vi "_PC_NS_Signal_Execution.vi"(0 "SysMsg":refnum<vi>, 1 "Network\nstream":refnum<vi>, 3 "Stop":refnum<vi>, 5 "# signal in NS":refnum<vi>, 11 "error in (no error)":errorcluster, 12 "Sig Queue":refnum<queue>, 14 "Conn_Bool":refnum<data-value>) -> ()   [LabVIEW 2018]
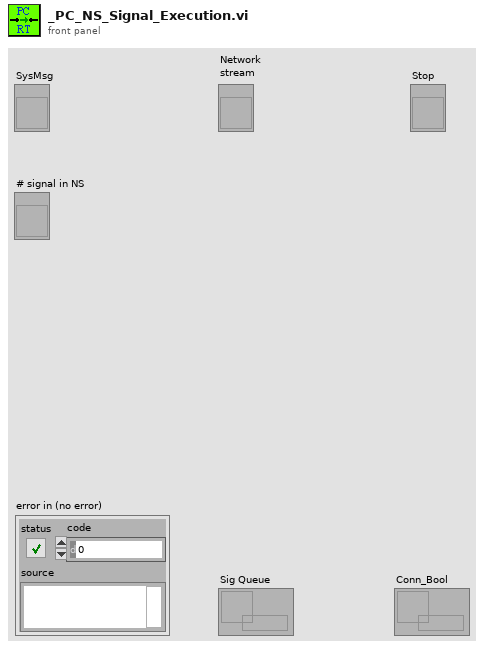
[diagram p1: front panel]
types:
  T1 = enum8{"Enabled", "Disabled", "Disabled and Grayed Out"}
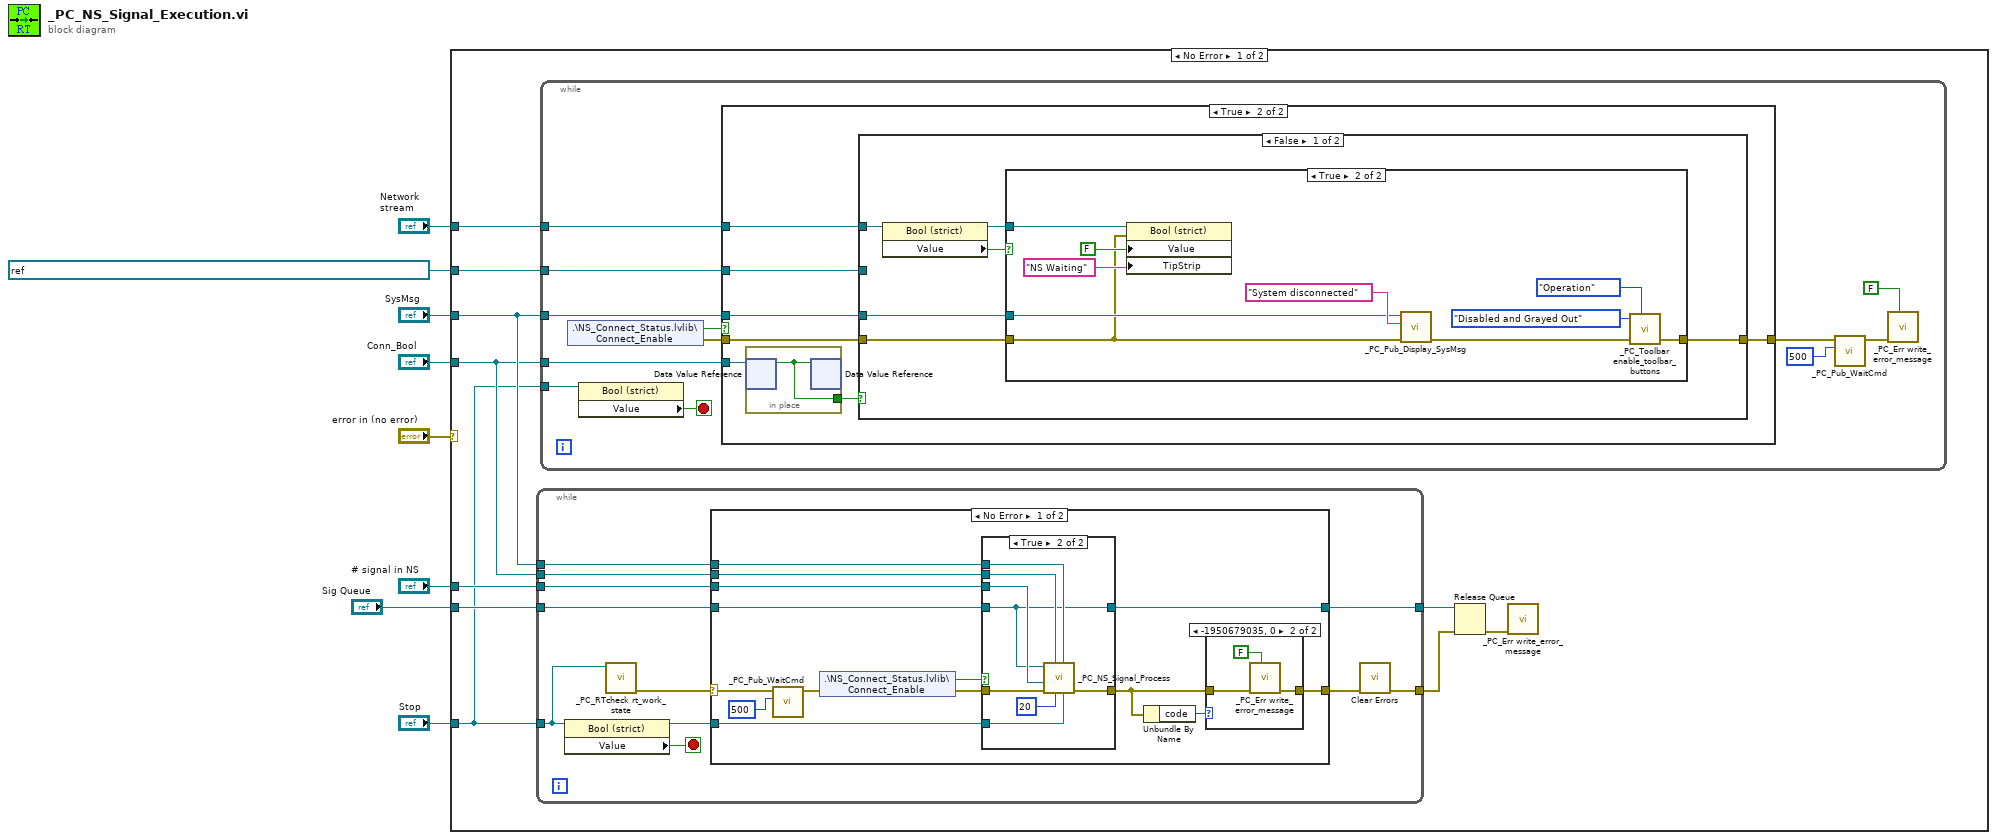
[diagram p0: block diagram]
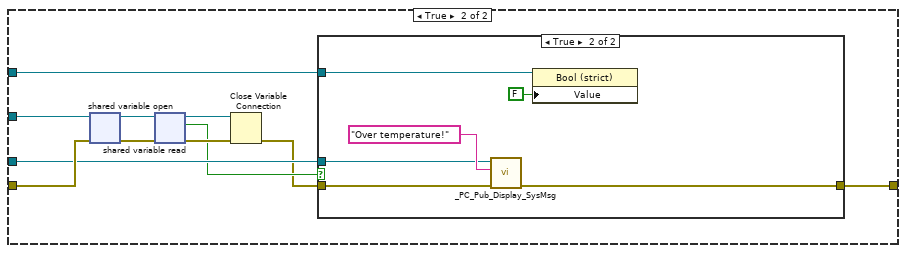
[diagram p4: hidden frame]
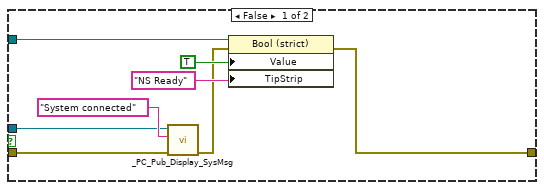
[diagram p5: hidden frame]
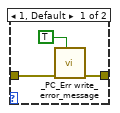
[diagram p6: hidden frame]
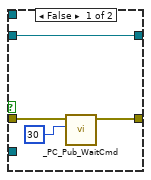
[diagram p7: hidden frame]
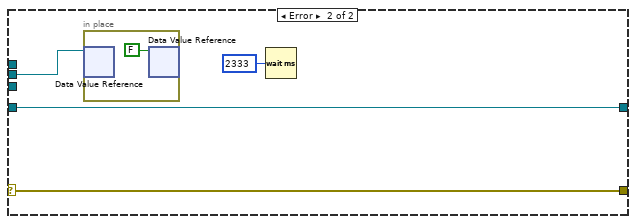
[diagram p8: hidden frame]
diagram:
  n1 = case shown="No Error" "error in (no error)" {
    tunnel: "# signal in NS" -> [w18 _]
    tunnel: "Network\nstream" -> [w17 _]
    tunnel: "SysMsg" -> [w16 _]
    tunnel: "Conn_Bool" -> [w15 _]
    tunnel: "Sig Queue" -> [w14 _]
    tunnel: refnum<k21> "ni.var.psp://NI-sbRIO/_RT_CtrlLoop_Safty_Variables/OverTemperature" ("shared variable refnum in") -> [w13 _]
    tunnel: "Stop" -> [w12 _]
    frame No Error {
      n2 = while {
        tunnel: w18 -> [w92]
        tunnel: w14 -> [w86]
        tunnel: w16 -> [w91]
        tunnel: w15 -> [w90]
        tunnel: w12 -> [w87]
        tunnel: [w85] -> w11
        tunnel: [w83] -> w10
        stop <- w89 stop-if-true
        n3 = property class="Bool (strict)"(reference=w87) -> (reference out=w82:refnum<vi>, "Value"=w89:bool)  [unwired: 1 in, 1 out]
        n4 = call "_PC_RTcheck rt_work_state.vi"("Stop"=w87) -> ("error out"=w88:errorcluster)  [unwired: 10 in]
        n5 = case shown="No Error" w88 {
          selector: w88 -> [w97 w126]
          tunnel: w92 -> [w106 _]
          tunnel: w91 -> [w103 _]
          tunnel: w90 -> [w102 w128]
          tunnel: [w94 w126] -> w84
          tunnel: w86 -> [w96 w125]
          tunnel: [w95 w125] -> w85
          tunnel: w82 -> [w93 _]
          frame No Error {
            n6 = call "_PC_Pub_WaitCmd.vi"("milliseconds to wait"=u32 500, "error in (no error)"=w97) -> ("error out"=w100:errorcluster)  [unwired: 9 in]
            n7 = shared-variable ".\\NS_Connect_Status.lvlib\\Connect_Enable"(error in=w100) -> (w104:bool, error out=w105:errorcluster)
            n8 = case shown="True" w104 {
              tunnel: w105 -> [w115 w123]
              tunnel: w106 -> [_ w122]
              tunnel: w96 -> [w113 w118]
              tunnel: [w114 w121] -> w98
              tunnel: w103 -> [_ w120]
              tunnel: w102 -> [_ w119]
              tunnel: [w113 w118] -> w95
              tunnel: w93 -> [_ w117]
              frame False {
                n9 = call "_PC_Pub_WaitCmd.vi"("milliseconds to wait"=u32 30, "error in (no error)"=w115) -> ("error out"=w114:errorcluster)  [unwired: 9 in]
              }
              frame True {
                n10 = call "_PC_NS_Signal_Process.vi"("Stop"=w117, "SysMsg"=w120, "Maximum Reader"=20, "Conn_Bool"=w119, "error in (no error)"=w123, "# signal in NS ref"=w122, "Sig Queue"=w118) -> ("error out"=w121:errorcluster)  [unwired: 4 in]
              }
            }
            n11 = Unbundle By Name(w98) -> ("code"=w99:i32)
            n12 = case shown="-1950679035, 0" w99 {
              tunnel: w98 -> [w108 w111]
              tunnel: [w107 w110] -> w94
              frame 1, Default {
                n13 = call "_PC_Err write_error_message.vi"("show msg( T )"=TRUE, "error in"=w108) -> ("error out"=w107:errorcluster)  [unwired: 9 in]
              }
              frame -1950679035, 0 {
                n14 = call "_PC_Err write_error_message.vi"("show msg( T )"=FALSE, "error in"=w111) -> ("error out"=w110:errorcluster)  [unwired: 9 in]
              }
            }
          }
          frame Error {
            n15 = in-place {
              n16 = in-place-dvr #1(w128) -> ()  [unwired: 2 out]
              n17 = in-place-dvr #1(FALSE ("data value")) -> ()  [unwired: 2 out]
            }
            n18 = Wait (ms)(milliseconds to wait=u32 2333) -> ()  [unwired: 1 out]
          }
        }
        n19 = call <vilib>:"Clear Errors.vi"("error in (no error)"=w84) -> ("error out"=w83:errorcluster)  [unwired: 5 in, 1 out]
      }
      n20 = while {
        tunnel: w16 -> [w29]
        tunnel: w17 -> [w28]
        tunnel: w15 -> [w27]
        tunnel: w13 -> [w22]
        tunnel: w12 -> [w20]
        stop <- w19 stop-if-true
        n21 = shared-variable ".\\NS_Connect_Status.lvlib\\Connect_Enable"() -> (w30:bool, error out=w26:errorcluster)  [unwired: 1 in]
        n22 = property class="Bool (strict)"(reference=w20) -> ("Value"=w19:bool)  [unwired: 1 in, 2 out]
        n23 = case shown="True" w30 {
          tunnel: w29 -> [_ w38]
          tunnel: w28 -> [_ w37]
          tunnel: [w31 w36] -> w24
          tunnel: w27 -> [_ w35]
          tunnel: w26 -> [w31 w33]
          tunnel: w22 -> [_ w32]
          frame False {
          }
          frame True {
            n24 = in-place {
              in-place-border: [w39] -> w34
              n25 = in-place-dvr #2(w35) -> (w39:bool)  [unwired: 1 out]
              n26 = in-place-dvr #2(w39) -> ()  [unwired: 2 out]
            }
            n27 = case shown="False" w34 {
              tunnel: w37 -> [w43 w63]
              tunnel: w33 -> [w45 w67]
              tunnel: [w44 w65] -> w36
              tunnel: w38 -> [w40 w66]
              tunnel: w32 -> [_ w64]
              frame False {
                n28 = property class="Bool (strict)"(reference=w43) -> (reference out=w41:refnum<vi>, "Value"=w42:bool)  [unwired: 1 in, 1 out]
                n29 = case shown="True" w42 {
                  tunnel: w45 -> [w46 w47]
                  tunnel: [w46 w48] -> w44
                  tunnel: w41 -> [_ w54]
                  tunnel: w40 -> [_ w49]
                  frame False {
                  }
                  frame True {
                    n30 = property class="Bool (strict)"(reference=w54, error in=w47, "Value"=FALSE, "TipStrip"="NS Waiting" ("Tip Strip")) -> ()  [unwired: 2 out]
                    n31 = call "_PC_Pub_Display_SysMsg.vi"("error in (no error)"=w47, "Msg String"="System disconnected" ("Msg in"), "SysMsg Ref In"=w49) -> ("error out"=w51:errorcluster)  [unwired: 7 in, 1 out]
                    n32 = call "_PC_Toolbar enable_toolbar_buttons.vi"("Disabled"=T1."Disabled and Grayed Out", "Function"=enum16{"Save reference", "Operation"}."Operation", "error in (no error)"=w51) -> ("error out"=w48:errorcluster)  [unwired: 6 in]
                  }
                }
              }
              frame True {
                n33 = shared-variable-open(w64, w67) -> (w59:refnum<k21>, w62:errorcluster)
                n34 = shared-variable-read(w59, w62) -> (w60:refnum<k21>, w61:errorcluster, w58:bool)
                n35 = Close Variable Connection(8:w61, 11:w60) -> (0:w57:errorcluster)
                n36 = case shown="True" w58 {
                  tunnel: w57 -> [w71 w80]
                  tunnel: [w68 w79] -> w65
                  tunnel: w66 -> [w70 w78]
                  tunnel: w63 -> [w69 w77]
                  frame False {
                    n37 = call "_PC_Pub_Display_SysMsg.vi"("error in (no error)"=w71, "Msg String"="System connected" ("Msg in"), "SysMsg Ref In"=w70) -> ("error out"=w72:errorcluster)  [unwired: 7 in, 1 out]
                    n38 = property class="Bool (strict)"(reference=w69, error in=w72, "Value"=TRUE, "TipStrip"="NS Ready" ("Tip Strip")) -> (error out=w68:errorcluster)  [unwired: 1 out]
                  }
                  frame True {
                    n39 = call "_PC_Pub_Display_SysMsg.vi"("error in (no error)"=w80, "Msg String"="Over temperature!" ("Msg in"), "SysMsg Ref In"=w78) -> ("error out"=w79:errorcluster)  [unwired: 7 in, 1 out]
                    n40 = property class="Bool (strict)"(reference=w77, "Value"=FALSE) -> ()  [unwired: 1 in, 2 out]
                  }
                }
              }
            }
          }
        }
        n41 = call "_PC_Pub_WaitCmd.vi"("milliseconds to wait"=u32 500, "error in (no error)"=w24) -> ("error out"=w23:errorcluster)  [unwired: 9 in]
        n42 = call "_PC_Err write_error_message.vi"("show msg( T )"=FALSE, "error in"=w23) -> ()  [unwired: 9 in, 1 out]
      }
      n43 = Release Queue(queue=w11, error in (no error)=w10) -> (error out=w9:errorcluster)  [unwired: 1 in, 2 out]
      n44 = call "_PC_Err write_error_message.vi"("error in"=w9) -> ()  [unwired: 10 in, 1 out]
    }
    frame Error {
    }
  }
